vi "Initialize Bus Controller.vi"(8 "error in (no error)":errorcluster, 9 "Next Available Buffer ID in":u16, 10 "Bus Controller":T1, 11 "Module Handle in":u32) -> (0 "error out":errorcluster, 1 "Next Available Buffer ID out":u16, 2 "BC Subaddress to Buffer ID Map":T5, 3 "Module Handle out":u32)   [LabVIEW 2020, in "AIM MIL-STD-1553 Engine.lvlib" / "Custom Device.lvlib"]
uses:
  Custom Device.lvlib
  Implementation/Shared Resources/BC Subaddress to Buffer ID Map.ctl
  Bus Controller Configuration.ctl
  Major Frame Configuration.ctl
  Minor Frame Configuration.ctl
  Message Configuration.ctl
  <instrlib>/_AIM MIL-STD-1553/AIM Controls/1553 Transfer Descriptor.ctl
  <vilib>/Utility/miscctls.llb/LVMapReplaceAction.ctl
  Implementation/Shared Resources/Shared Resources.lvclass
  Hardware API/AIM MIL-STD-1553 Hardware API.lvlib
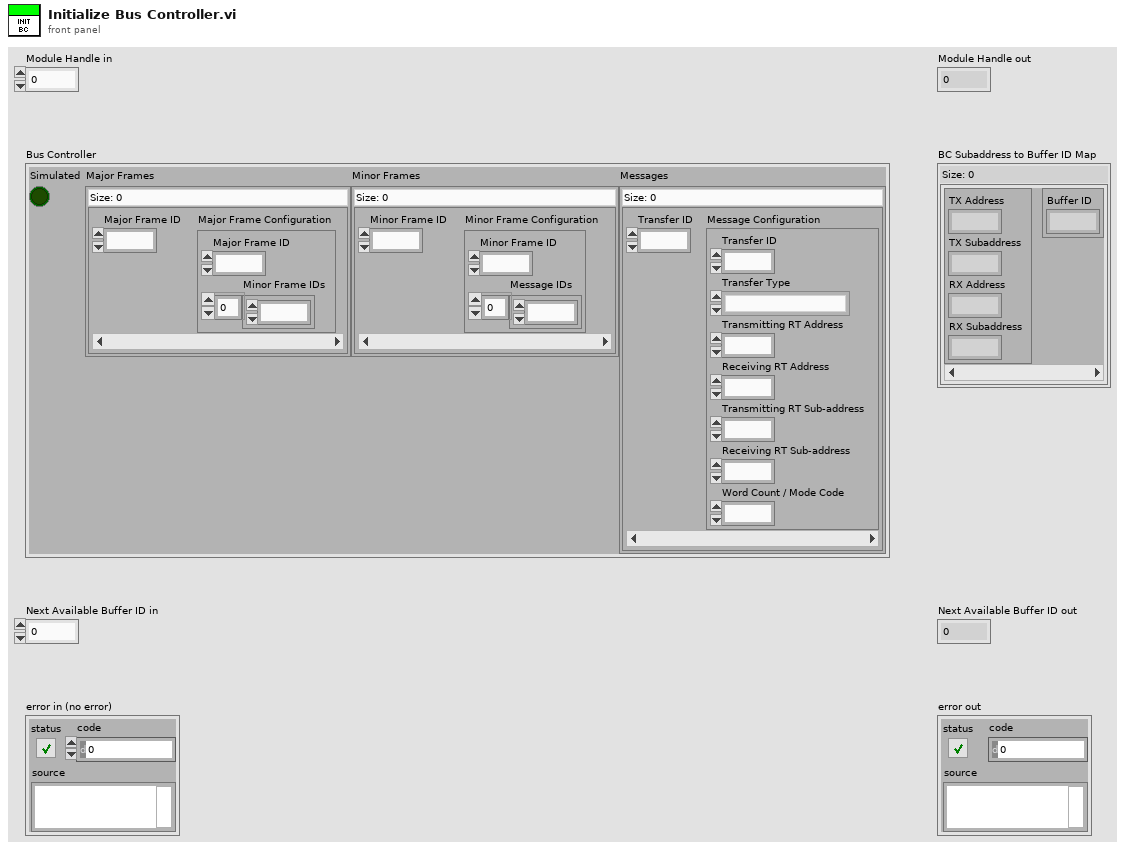
[diagram p1: front panel]
types:
  T1 = typedef "AIM MIL-STD-1553 Engine.lvlib/Custom Device.lvlib/Bus Controller Configuration.ctl" = cluster{"Simulated":bool, "Major Frames":map{u8, T2}, "Minor Frames":map{u8, T3}, "Messages":map{u16, T4}}
  T2 = typedef "AIM MIL-STD-1553 Engine.lvlib/Custom Device.lvlib/Major Frame Configuration.ctl" = cluster{"Major Frame ID":u8, "Minor Frame IDs":u8[]}
  T3 = typedef "AIM MIL-STD-1553 Engine.lvlib/Custom Device.lvlib/Minor Frame Configuration.ctl" = cluster{"Minor Frame ID":u8, "Message IDs":u16[]}
  T4 = typedef "AIM MIL-STD-1553 Engine.lvlib/Custom Device.lvlib/Message Configuration.ctl" = cluster{"Transfer ID":u16, "Transfer Type":enum16{"BC to RT transfer", "RT to BC transfer", "RT to RT transfer"}, "Transmitting RT Address":u8, "Receiving RT Address":u8, "Transmitting RT Sub-address":u8, "Receiving RT Sub-address":u8, "Word Count / Mode Code":u8}
  T5 = typedef "AIM MIL-STD-1553 Engine.lvlib/Implementation.lvlib/Shared Resources.lvclass/BC Subaddress to Buffer ID Map.ctl" = map{cluster{"TX Address":u8, "TX Subaddress":u8, "RX Address":u8, "RX Subaddress":u8}, cluster{"Buffer ID":u16}}
  T6 = typedef "1553 Transfer Descriptor.ctl" = cluster{"Transfer ID":u16, "Buffer Header ID":u16, "Transfer Type":enum16{"BC to RT transfer", "RT to BC transfer", "RT to RT transfer"}, "Bus":enum16{"primary", "secondary"}, "Transmitting RT Address":u8, "Receiving RT Address":u8, "Transmitting RT Sub-address":u8, "Receiving RT Sub-address":u8, "Word Count / Mode Code":u8, "Interrupt Control":enum16{"none", "on end of transfer", "on transfer error", "on status word exception"}, "Halt Control":enum16{"none", "on transfer error", "on status word exception", "on both", "on any interrupt"}, "Retry Control":enum16{"disable", "enable", "keep bus at next transmit", "alternate bus on next transmit"}, "Expected Response":enum16{"automatic", "no status word 1", "no status word 2"}, "Gap Mode":enum16{"delay", "standard", "fast"}, "Transfer Wait Time":u16}
  T7 = typedef "LVMapReplaceAction.ctl" = enum32{"Modify Entry only if found", "Add or Modify Entry", "Delete Entry"}
  T8 = enum16{"BC to RT transfer", "RT to BC transfer", "RT to RT transfer"}
  T9 = cluster{"Transmitting RT Address":u8, "Transmitting RT Sub-address":u8, "Receiving RT Address":u8, "Receiving RT Sub-address":u8}
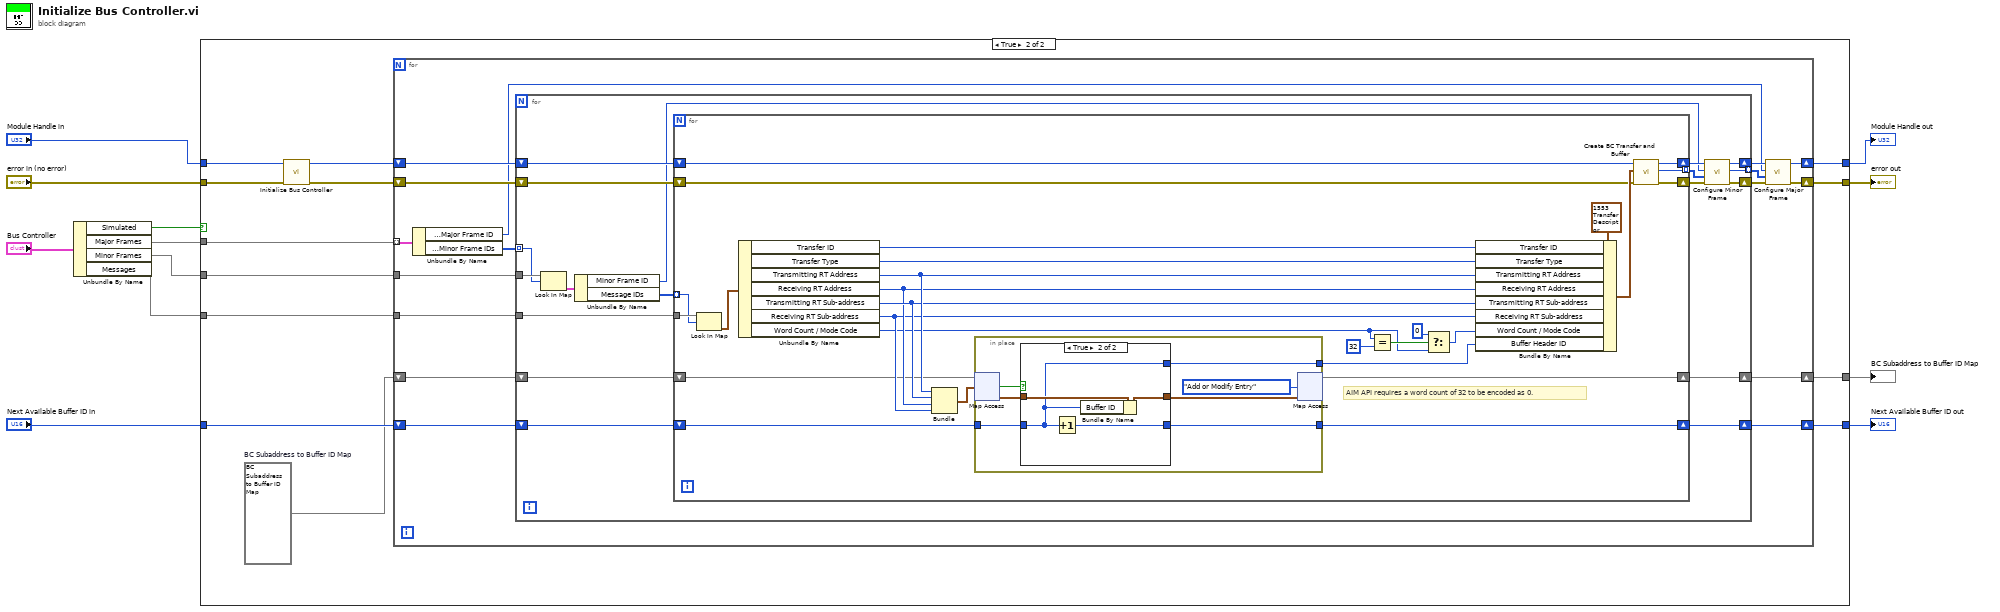
[diagram p0: block diagram]
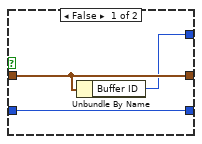
[diagram p3: hidden frame]
diagram:
  n1 = Unbundle By Name("Bus Controller") -> ("Simulated"=w7:bool, "Major Frames"=w1:map{u8, T2}, "Minor Frames"=w2:map{u8, T3}, "Messages"=w3:map{u16, T4})
  n2 = case shown="True" w7 {
    tunnel: w1 -> [_ w28]
    tunnel: w2 -> [_ w27]
    tunnel: w3 -> [_ w26]
    tunnel: "Module Handle in" -> [w14 w21]
    tunnel: "error in (no error)" -> [w13 w20]
    tunnel: "Next Available Buffer ID in" -> [w15 w25]
    tunnel: [w14 w24] -> w5
    tunnel: [w13 w23] -> w6
    tunnel: [w15 w22] -> w11
    tunnel: [_ w17] -> w12
    frame False {
    }
    frame True {
      w16 = T5 {}  # BC Subaddress to Buffer ID Map
      n3 = call "Initialize Bus Controller.vi"("Error In"=w20, "Module Handle"=w21) -> ("Error Out"=w18:errorcluster, "Module Handle out"=w19:u32)  [unwired: 8 in]
      n4 = for {
        tunnel: w28 -> [w44] mode=indexing
        tunnel: w27 -> [w42]
        tunnel: w26 -> [w41]
        shift-right: [w36] -> w23
        shift-left: w18 -> [w39]
        shift-right: [w35] -> w24
        shift-left: w19 -> [w40]
        shift-right: [w31] -> w22
        shift-left: w25 -> [w32]
        shift-right: [w29] -> w17
        shift-left: w16 -> [w30]
        n5 = Unbundle By Name(w44) -> ("Major Frame Configuration.Major Frame ID"=w34:u8, "Major Frame Configuration.Minor Frame IDs"=w43:u8[])
        n6 = for {
          tunnel: w43 -> [w61] mode=indexing
          tunnel: w42 -> [w62]
          tunnel: w41 -> [w58]
          shift-right: [w54] -> w38
          shift-left: w39 -> [w56]
          shift-right: [w52] -> w37
          shift-left: w40 -> [w57]
          tunnel: [w50] -> w33 mode=indexing
          shift-right: [w47] -> w31
          shift-left: w32 -> [w48]
          shift-right: [w45] -> w29
          shift-left: w30 -> [w46]
          n7 = Look In Map(map=w62, key=w61) -> (value=w60:T3)  [unwired: 1 in, 1 out]
          n8 = Unbundle By Name(w60) -> ("Minor Frame ID"=w51:u8, "Message IDs"=w59:u16[])
          n9 = for {
            tunnel: w59 -> [w86] mode=indexing
            tunnel: w58 -> [w87]
            shift-right: [w82] -> w55
            shift-left: w56 -> [w83]
            shift-right: [w81] -> w53
            shift-left: w57 -> [w84]
            tunnel: [w80] -> w49 mode=indexing
            shift-right: [w77] -> w47
            shift-left: w48 -> [w78]
            shift-right: [w70] -> w45
            shift-left: w46 -> [w71]
            # "AIM API requires a word count of 32 to be encoded as 0."
            n10 = Look In Map(map=w87, key=w86) -> (value=w85:T4)  [unwired: 1 in, 1 out]
            n11 = Unbundle By Name(w85) -> ("Transfer ID"=w79:u16, "Transfer Type"=w76:T8, "Transmitting RT Address"=w75:u8, "Receiving RT Address"=w73:u8, "Transmitting RT Sub-address"=w74:u8, "Receiving RT Sub-address"=w72:u8, "Word Count / Mode Code"=w63:u8)
            n12 = Bundle("Transmitting RT Address"=w75, "Transmitting RT Sub-address"=w74, "Receiving RT Address"=w73, "Receiving RT Sub-address"=w72) -> (w69:T9)  [unwired: 1 in]
            n13 = in-place {
              in-place-border: w78 -> [w95]
              in-place-border: [w93] -> w77
              in-place-border: [w90] -> w68
              n14 = in-place-map #1(w71, w69) -> (w92:cluster{"Buffer ID":u16}, w96:bool)  [unwired: 1 in]
              n15 = case shown="True" w96 {
                tunnel: w95 -> [w99 w100]
                tunnel: [w98 w101] -> w91
                tunnel: [w99 w103] -> w93
                tunnel: w92 -> [w98 w102]
                tunnel: [w97 w100] -> w90
                frame False {
                  n16 = Unbundle By Name(w98) -> ("Buffer ID"=w97:u16)
                }
                frame True {
                  n17 = Increment(x=w100) -> (x+1=w103:u16)
                  n18 = Bundle By Name(cluster=w102, "Buffer ID"=w100) -> (w101:cluster{"Buffer ID":u16})
                }
              }
              n19 = in-place-map #1(w91, LVMapReplaceAction."Add or Modify Entry" ("action")) -> (w70:T5)  [unwired: 2 out]
            }
            n20 = Equal?(x=w63, y=u8 32) -> (x = y?=w66:bool)
            n21 = Select(t=u8 0, s=w66, f=w63) -> (s? t:f=w64:u8)
            n22 = Bundle By Name(cluster=T6 {"Transfer ID"=0, "Buffer Header ID"=0, "Transfer Type"=enum."BC to RT transfer", "Bus"=enum."primary", "Transmitting RT Address"=0, "Receiving RT Address"=0, "Transmitting RT Sub-address"=0, "Receiving RT Sub-address"=0, "Word Count / Mode Code"=0, "Interrupt Control"=enum."none", "Halt Control"=enum."none", "Retry Control"=enum."disable", "Expected Response"=enum."automatic", "Gap Mode"=enum."delay", "Transfer Wait Time"=0} ("BC Transfer Descriptor"), "Transfer ID"=w79, "Transfer Type"=w76, "Transmitting RT Address"=w75, "Receiving RT Address"=w73, "Transmitting RT Sub-address"=w74, "Receiving RT Sub-address"=w72, "Word Count / Mode Code"=w64, "Buffer Header ID"=w68) -> (w88:T6)
            n23 = call "Create BC Transfer and Buffer.vi"("Error In"=w83, "BC Transfer Descriptor"=w88, "Module Handle"=w84) -> ("Error Out"=w82:errorcluster, "Transfer ID out"=w80:u16, "Module Handle out"=w81:u32)  [unwired: 6 in]
          }
          n24 = call "Configure Minor Frame.vi"("Error In (none)"=w55, "Transfer IDs"=w49, "Minor Frame ID"=w51, "Module Handle"=w53) -> ("Error Out"=w54:errorcluster, "Minor Frame ID out"=w50:u8, "Module Handle out"=w52:u32)  [unwired: 5 in]
        }
        n25 = call "Configure Major Frame.vi"("Error In (none)"=w38, "Minor Frame IDs"=w33, "Major Frame ID"=w34, "Module Handle"=w37) -> ("Error Out"=w36:errorcluster, "Module Handle out"=w35:u32)  [unwired: 5 in, 1 out]
      }
    }
  }
  "BC Subaddress to Buffer ID Map" <- w12
  "Next Available Buffer ID out" <- w11
  "error out" <- w6
  "Module Handle out" <- w5
